vi "Sum.vi"(6 "LabVIEW Web Service Request":refnum<class "Web Request.lvclass">, 9 "NEWNUM":dbl, 10 "MODE":string="INPUT") -> (3 "SUM 2":dbl)   [LabVIEW 2016]
uses:
  <vilib>/wsapi/Web Request.lvclass
  <vilib>/Utility/xml.llb/Read From XML File(string).vi
  <vilib>/Utility/xml.llb/Write to XML File(string).vi
panel:
  out "value":string="INPUT"
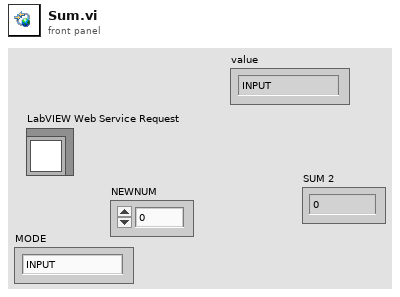
[diagram p1: front panel]
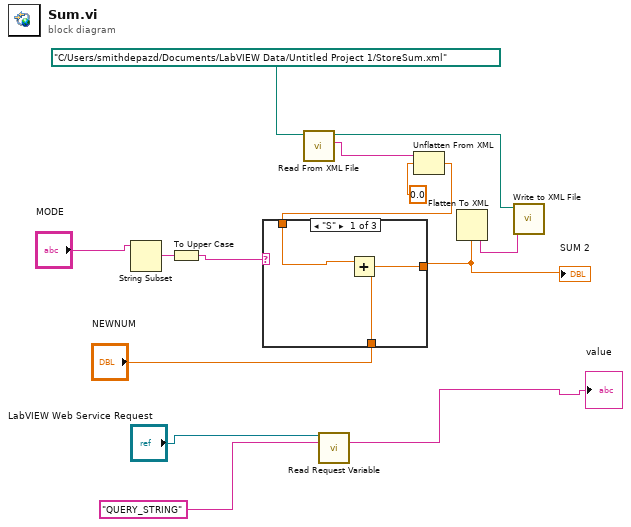
[diagram p0: block diagram]
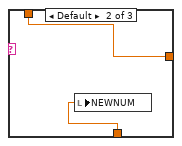
[diagram p2: hidden frame]
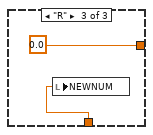
[diagram p3: hidden frame]
diagram:
  n1 = String Subset(string="MODE") -> (substring=w8:string)  [unwired: 2 in]
  n2 = To Upper Case(1:w8) -> (0:w7:string)
  n3 = call-poly <vilib>:"Read From XML File.vi"("XML File Path"=path "C:/Users/smithdepazd/Documents/LabVIEW Data/Untitled Project 1/StoreSum.xml") -> ("XML Elements"=w12:string, "XML File Path(duplicate)"=w1:path)  [unwired: 8 in, 1 out]
  n4 = call <vilib>:"Read Request Variable.vi"("LabVIEW Web Service Request"="LabVIEW Web Service Request", "variable name"="QUERY_STRING") -> ("value"=→"value":string)  [unwired: 11 in, 2 out]
  n5 = Unflatten From XML(xml string=w12, type=0.0) -> (value=w3:dbl)  [unwired: 1 in, 1 out]
  n6 = case shown="\"S\"" w7 {
    tunnel: [w17 w18 0.0] -> w2
    tunnel: "NEWNUM" -> [w16 w19 w20]
    tunnel: w3 -> [w15 w18 _]
    frame "S" {
      n7 = Add(x=w15, y=w16) -> (x+y=w17:dbl)
    }
    frame Default {
      n8 = local write "NEWNUM"(w19) -> ()
    }
    frame "R" {
      n9 = local write "NEWNUM"(w20) -> ()
    }
  }
  "SUM 2" <- w2
  n10 = Flatten To XML(anything=w2) -> (xml string=w10:string)
  n11 = call-poly <vilib>:"Write to XML File.vi"("XML Input"=w10, "XML File Path"=w1) -> ()  [unwired: 7 in, 3 out]
